vi "Update UI Logs Display.vi"(8 "error in (no error)":errorcluster, 10 "Display References":refnum<vi>[](array[refnum]), 11 "Log Array Subset":T1[](array[typedef])) -> (0 "error out":errorcluster)   [LabVIEW 2019]
uses:
  Controls/Log.ctl
  Controls/Log State.ctl
  Controls/Log Row.ctl
  Controls/Log Row Download State Indicator.ctl
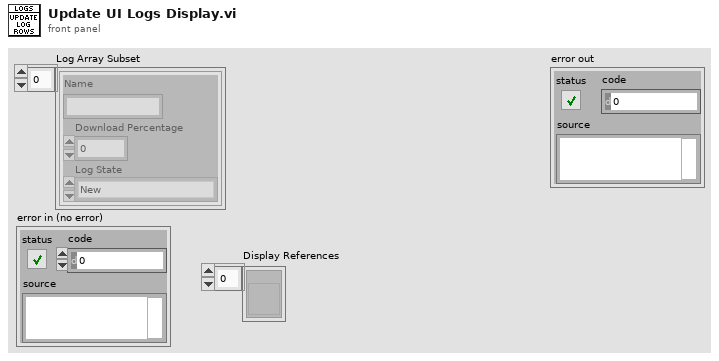
[diagram p1: front panel]
types:
  T1 = typedef "Log.ctl" = cluster{"Name":string, "Download Percentage":dbl, "Log State":T2}
  T2 = typedef "Log State.ctl" = enum16{"New", "Downloading", "Downloaded"}
  T3 = typedef "Log Row.ctl" = cluster{"Day":string, "Date":string, "Log Row Download":T4, "Download Progress":u8, "Log Progress":dbl}
  T4 = typedef "Log Row Download State Indicator.ctl" = u16
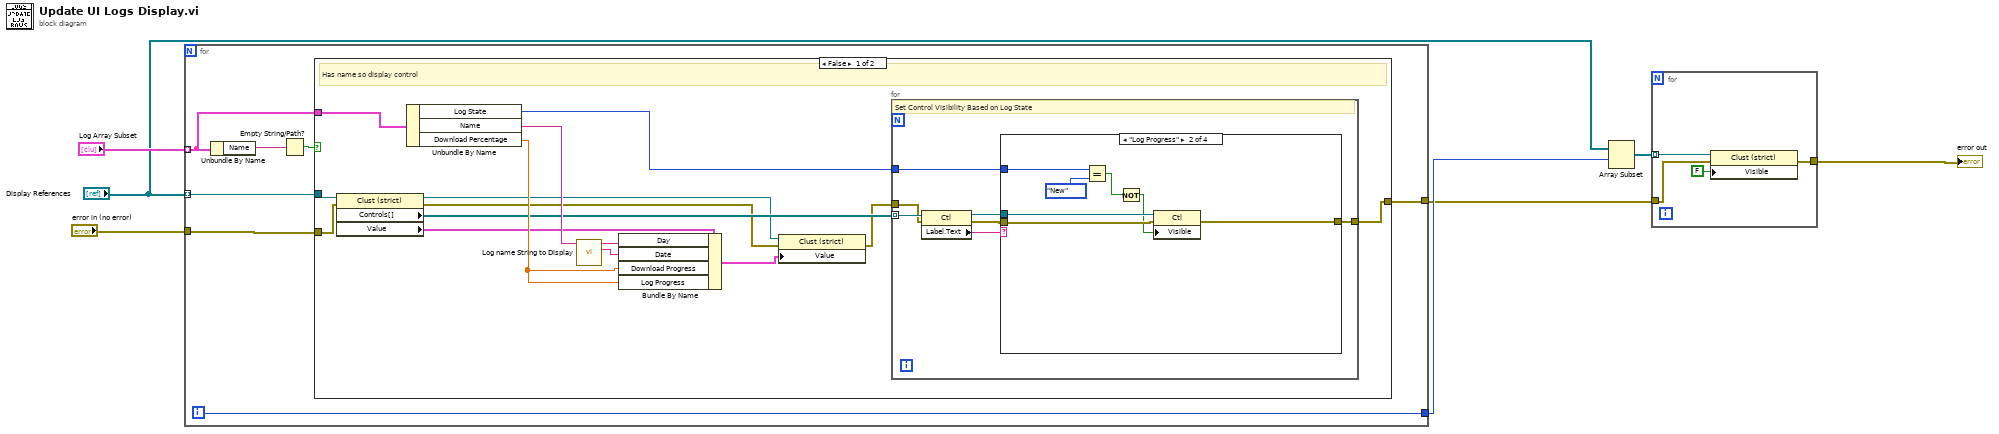
[diagram p0: block diagram]
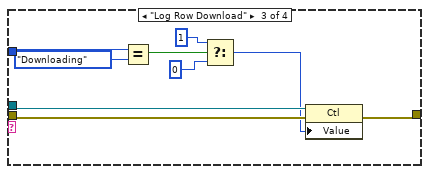
[diagram p3: hidden frame]
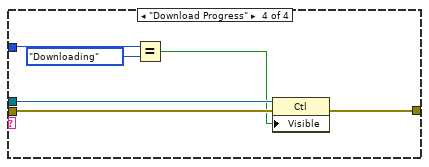
[diagram p4: hidden frame]
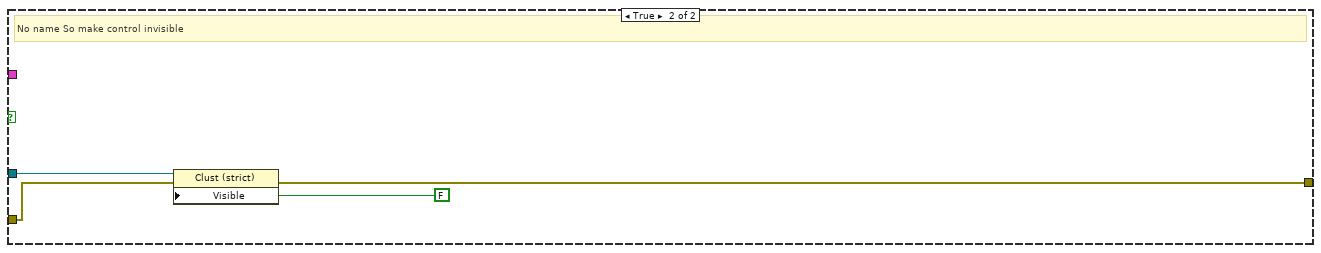
[diagram p5: hidden frame]
diagram:
  n1 = for {
    tunnel: "Log Array Subset" -> [w9] mode=indexing
    tunnel: "Display References" -> [w13] mode=indexing
    tunnel: "error in (no error)" -> [w11]
    tunnel: [w10] -> w2
    tunnel: [w8] -> w4
    i -> [w8]
    n2 = Unbundle By Name(w9) -> ("Name"=w14:string)
    n3 = Empty String/Path?(string/path=w14) -> (empty?=w12:bool)
    n4 = case shown="False" w12 {
      tunnel: w13 -> [w29 w63]
      tunnel: w11 -> [w28 w61]
      tunnel: [w19 w60] -> w10
      tunnel: w9 -> [w27 _]
      frame False {
        # "Has name so display control"
        n5 = property class="Clust (strict)"(reference=w29, error in=w28) -> (reference out=w18:refnum<vi>, error out=w16:errorcluster, "Controls[]"=w21:refnum<vi>[], "Value"=w22:T3)
        n6 = Unbundle By Name(w27) -> ("Log State"=w20:T2, "Name"=w26:string, "Download Percentage"=w23:dbl)
        n7 = call "Log name String to Display.vi"("Log Name"=w26) -> ("Date"=w24:string, "Day"=w25:string)  [unwired: 9 in]
        n8 = Bundle By Name(cluster=w22, "Day"=w25, "Date"=w24, "Download Progress"=w23, "Log Progress"=w23) -> (w17:T3)
        n9 = property class="Clust (strict)"(reference=w18, error in=w16, "Value"=w17) -> (error out=w15:errorcluster)  [unwired: 1 out]
        n10 = for {
          tunnel: w21 -> [w36] mode=indexing
          tunnel: w15 -> [w35]
          tunnel: w20 -> [w32]
          tunnel: [w30] -> w19
          # "Set Control Visibility Based on Log State"
          n11 = property class="Ctl"(reference=w36, error in=w35) -> (reference out=w33:refnum<vi>, error out=w31:errorcluster, "Label.Text"=w34:string)
          n12 = case shown="\"Log Progress\"" w34 {
            tunnel: w33 -> [_ w42 w48 w56]
            tunnel: w32 -> [_ w44 w53 w59]
            tunnel: w31 -> [w37 w41 w46 w55]
            tunnel: [w37 w40 w47 w57] -> w30
            frame Default {
            }
            frame "Log Progress" {
              n13 = Equal?(x=w44, y=Log_State."New") -> (x = y?=w39:bool)
              n14 = Not(x=w39) -> (.not. x?=w38:bool)
              n15 = property class="Ctl"(reference=w42, error in=w41, "Visible"=w38) -> (error out=w40:errorcluster)  [unwired: 1 out]
            }
            frame "Log Row Download" {
              n16 = Equal?(x=w53, y=Log_State."Downloading") -> (x = y?=w51:bool)
              n17 = Select(t=1, s=w51, f=0) -> (s? t:f=w45:i32)
              n18 = property class="Ctl"(reference=w48, error in=w46, "Value"=w45) -> (error out=w47:errorcluster)  [unwired: 1 out]
            }
            frame "Download Progress" {
              n19 = Equal?(x=w59, y=Log_State."Downloading") -> (x = y?=w54:bool)
              n20 = property class="Ctl"(reference=w56, error in=w55, "Visible"=w54) -> (error out=w57:errorcluster)  [unwired: 1 out]
            }
          }
        }
      }
      frame True {
        # "No name So make control invisible"
        n21 = property class="Clust (strict)"(reference=w63, error in=w61, "Visible"=FALSE) -> (error out=w60:errorcluster)  [unwired: 1 out]
      }
    }
  }
  n22 = Array Subset(array="Display References", index=w4) -> (w3:refnum<vi>[])  [unwired: 1 in]
  n23 = for {
    tunnel: w3 -> [w67] mode=indexing
    tunnel: w2 -> [w65]
    tunnel: [w64] -> w1
    n24 = property class="Clust (strict)"(reference=w67, error in=w65, "Visible"=FALSE) -> (error out=w64:errorcluster)  [unwired: 1 out]
  }
  "error out" <- w1
